vi "AVS_Measure.vi"(0 "a_hDevice":i32, 7 "a_hWnd":i32, 11 "a_Nmsr":i16) -> (4 "Output Value":i32)   [LabVIEW 2013, in "Avantes Spectrometer Functions.lvlib"]
uses:
  Avantes Spectrometer Functions.lvlib
  AvantesSpectrometer2/polling_mc/AS5216.dll
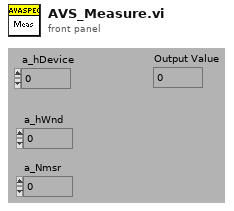
[diagram p1: front panel]
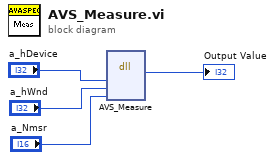
[diagram p0: block diagram]
diagram:
  n1 = dll-call lib="C:/Users/dhstuart/Dropbox/CLTC/AvantesSpectrometer2/polling_mc/AS5216.dll" fn="AVS_Measure"("a_hDevice"="a_hDevice", "a_hWnd"="a_hWnd", "a_Nmsr"="a_Nmsr") -> (→"Output Value":i32)  [unwired: 6 in, 2 out]
